vi "FormCalibra5.vi"() -> ()   [LabVIEW 2014]
uses:
  testMachine.ctl
  mainMachine.ctl
  <vilib>/Analysis/baseanly.llb/Mean (DBL).vi
  <vilib>/express/express shared/transition.llb/Dynamic To Waveform Array.vi
  <vilib>/express/express signal manip/GetorSetDDTAttributes/Set DDT Attributes/SetT0.vi
  <vilib>/express/express shared/transition.llb/Waveform Array To Dynamic.vi
  <vilib>/express/express signal manip/GetorSetDDTAttributes/Set DDT Attributes/Set DDT Properties.xnode
  <vilib>/Analysis/NI_AALBase.lvlib
  <resource>/objmgr/daqmx.rc
panel:
  out "deviceName":tag
  out "editTotalWaitLimit":u8
  out "editCountWaitLimit":u8
  out "ledWaitState":bool caption="Wait State"
  out "sliderWaitUpperTime":u8(slide) max=50 scale=0.0..50.0
  out "slideWaitLowerTime":u8(slide) max=30 scale=0.0..30.0
  out "slideWaitTime":u8(slide) scale=0.0..150.0
  out "labelTestTime":string caption="Tempo total de ensaio"
  in  "buttonAcquisition":bool
  in  "editSetWaitTime":u8 caption="Tempo entre ciclos (s)" step=1 format="%0d"
  in  "stop":bool
  out "error out":errorcluster
  out "ledAcquireState":bool caption="Acquire State"
  out "editTotalLowerLimit":u8
  out "editCountLowerLimit":u8
  out "editTotalUpperLimit":u8
  out "editCountUpperLimit":u8
  out "ledEnsaio 3":bool
  out "ledBrakeState":bool caption="Brake State"
  out "ledExitState":bool caption="Exit State"
  out "ledMotorState":bool caption="Motor State"
  out "ledInit2State":bool caption="Init State"
  out "ledBlockState":bool caption="Block State"
  out "ledRunningState":bool caption="Running State"
  out "ledReadyState":bool caption="Ready State"
  out "ledInitState":bool caption="Init State"
  out "mainMachine":T1
  out "testMachine":T2=enum."finish"
  in  "editSetPathToFile":path
  in  "buttonStop":bool
  in  "buttonStart":bool
  out "graphForce":dynamicdata(graph)
  in  "editOffsetForce":dbl caption="Tara" min=0.0 max=100.0 step=0.1
  in  "editSetForce":dbl caption="Fator de conversão"
  out "editForce":dbl caption="Força (Kgf)" format="%#_4f"
  out "graphSpeed":dynamicdata(graph)
  in  "editSetSpeed":dbl caption="Fator de conversão"
  out "editSpeed":dbl caption="Velocidade (km/h)" format="%#_4f"
  out "editEngineSpeed":dbl caption="Rotação (RPM)" format="%#_4f"
  in  "buttonMotor":bool
  in  "buttonBrake":bool
  in  "editSetWaitLowerTime":u8 caption="Tempo de espera (s)"
  in  "editSetWaitUpperTime":u8=3 caption="Tempo de espera (s)"
  in  "editSetNumberOfCycles":u16 caption="Número de ciclos" max=999 step=1 format="%0d"
  in  "editSetLowerLimit":u32 caption="Limite inferior (km/h)"
  in  "editSetUpperLimit":u32 caption="Limite superior (km/h)"
  out "editTempB":dbl caption="Temperatura B (ºC)"
  out "editTempA":dbl caption="Temperatura A (ºC)"
  in  "editSetTempRef":dbl caption="Offset referência" step=0.01 format="%#_2f"
  out "editTempRef":dbl caption="Referência (ºC)"
  out "ledMotor":bool
  out "ledBrake":bool
  out "ledEnsaio":bool
  out "labelTotalCycle":string
  out "labelCurrentCycle":string
  out "labelSystemTitle":string
  in  "editCurrCycleCtr":u32
  in  "velocidade 2":u32
  out "velocidade":u32
  # "Bancada de Frenagem - Ensaio"
  # "Ensaio"
  # "Temperatura"
  # "Rotação"
  # "Célula de Carga"
  # "Configurações do ensaio"
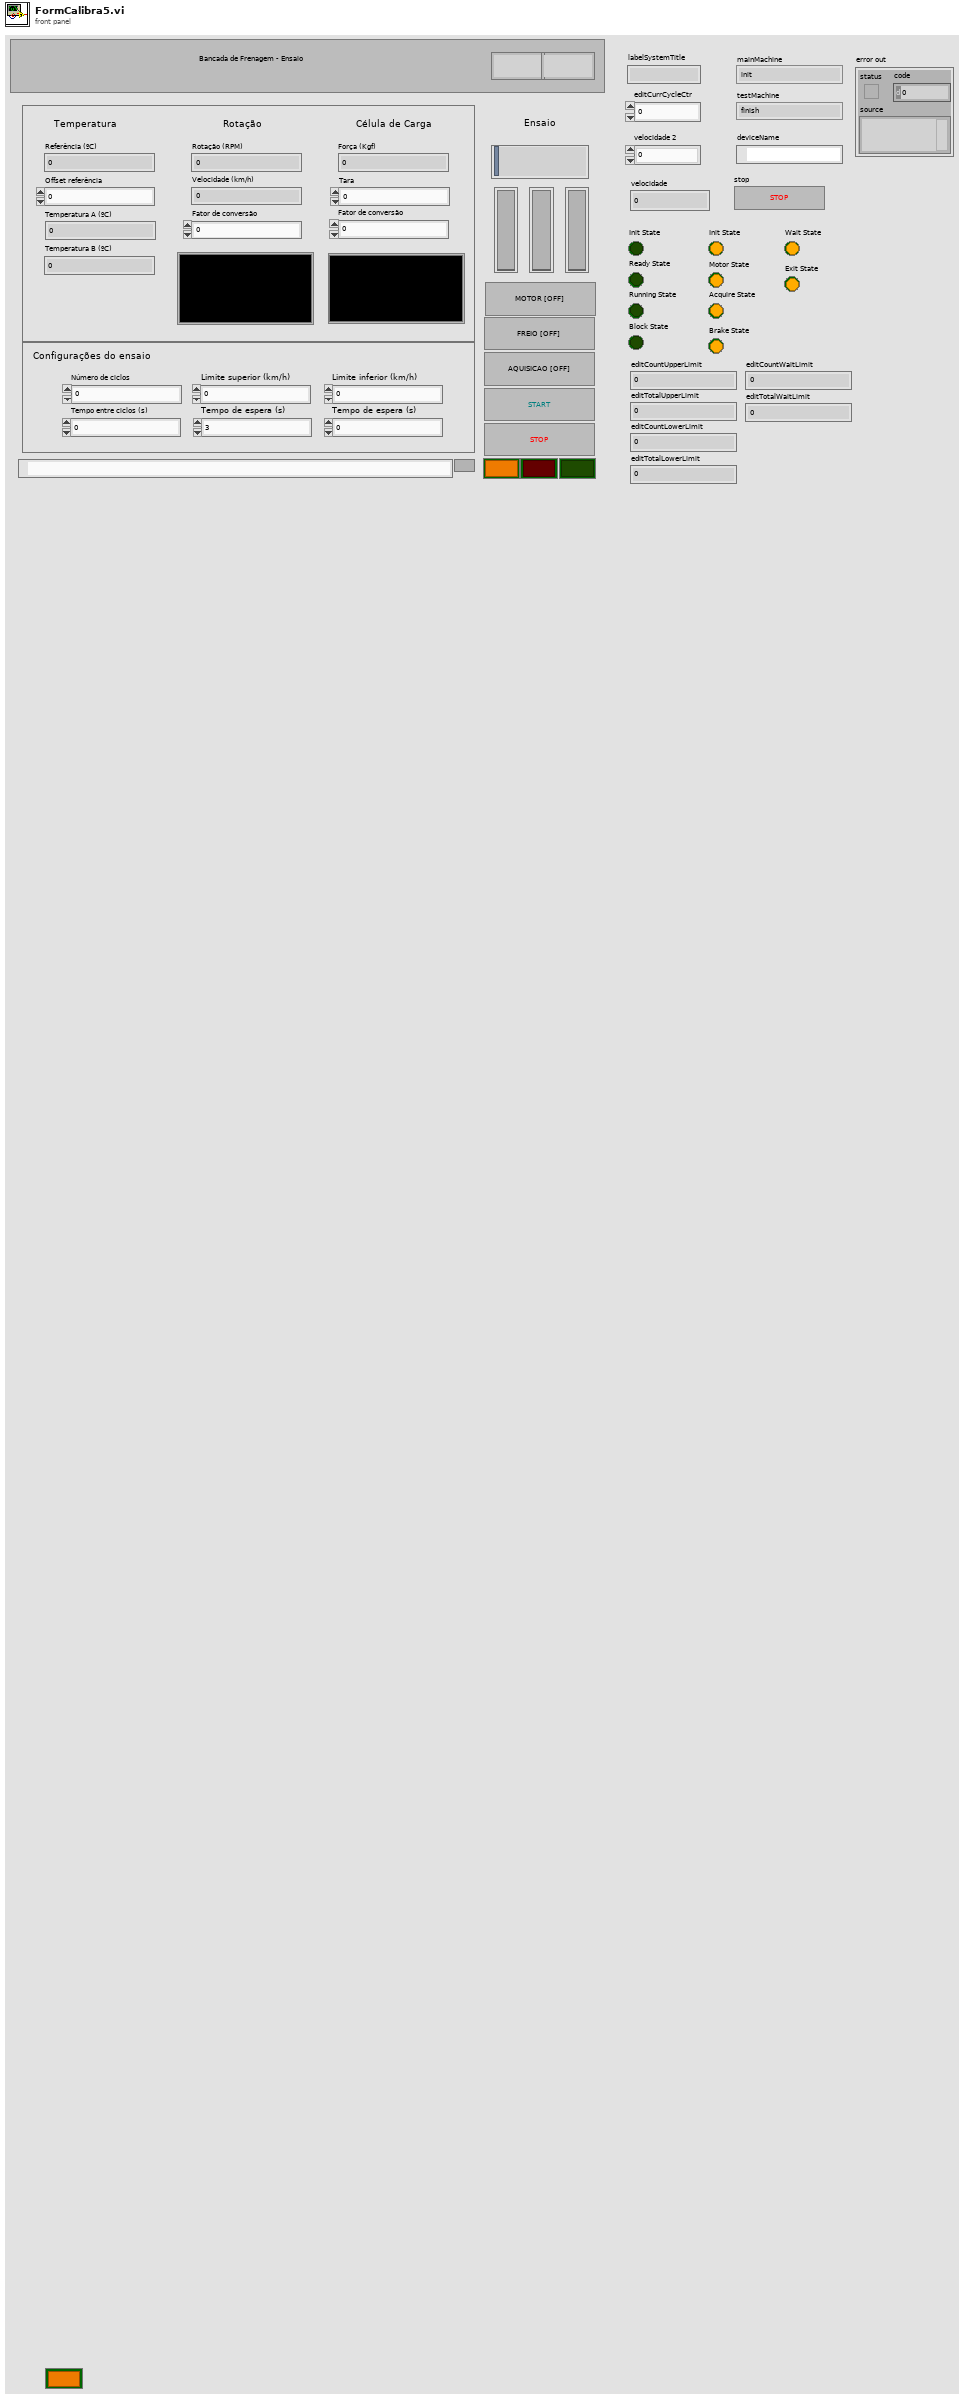
[diagram p1: front panel]
types:
  T1 = typedef "mainMachine.ctl" = enum16{"init", "ready", "running", "blocked", "finish"}
  T2 = typedef "testMachine.ctl" = enum16{"init", "motor", "motor acquire", "brake", "brake acquire", "wait ", "finish", "exit"}
  T3 = enum8{"Enabled", "Disabled", "Disabled and Grayed Out"}
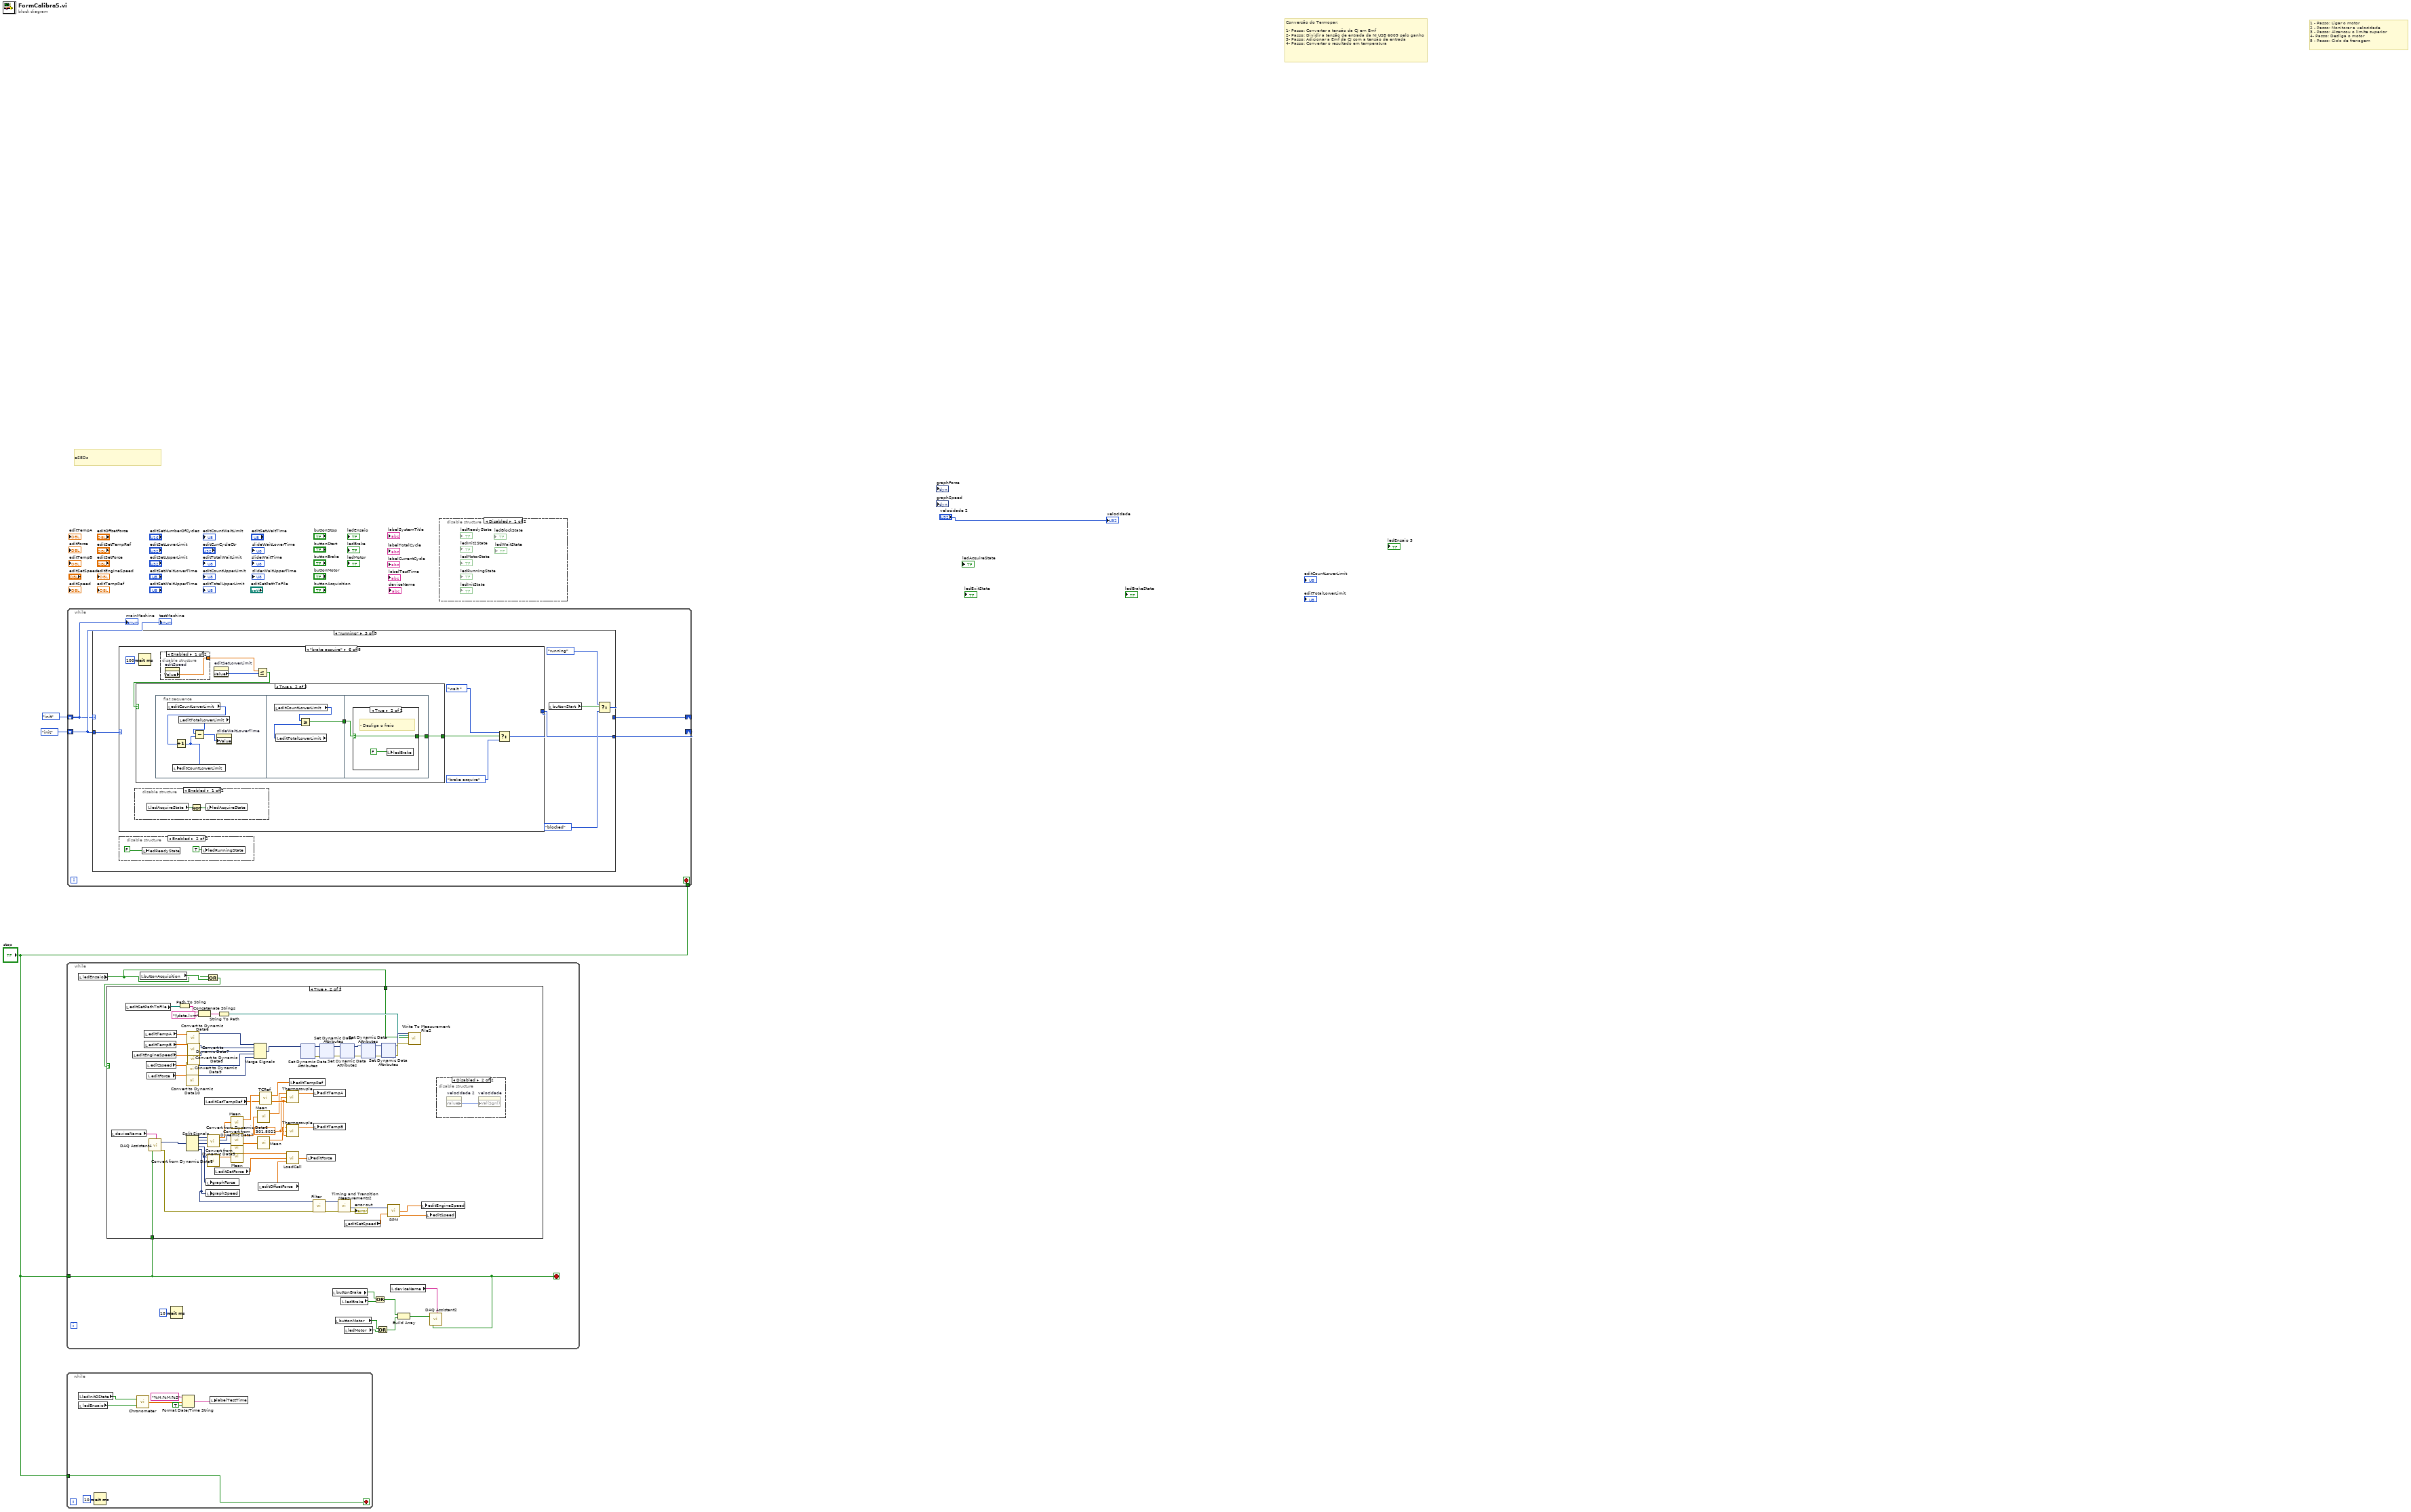
[diagram p0: block diagram]
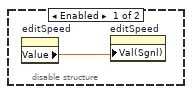
[diagram p4: hidden frame]
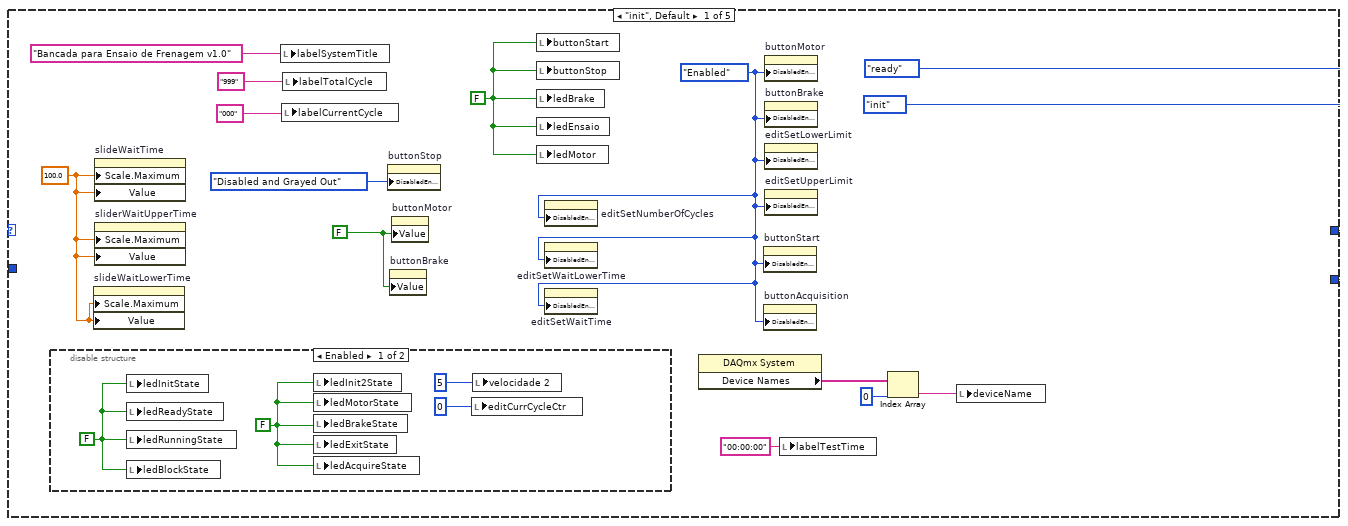
[diagram p5: hidden frame]
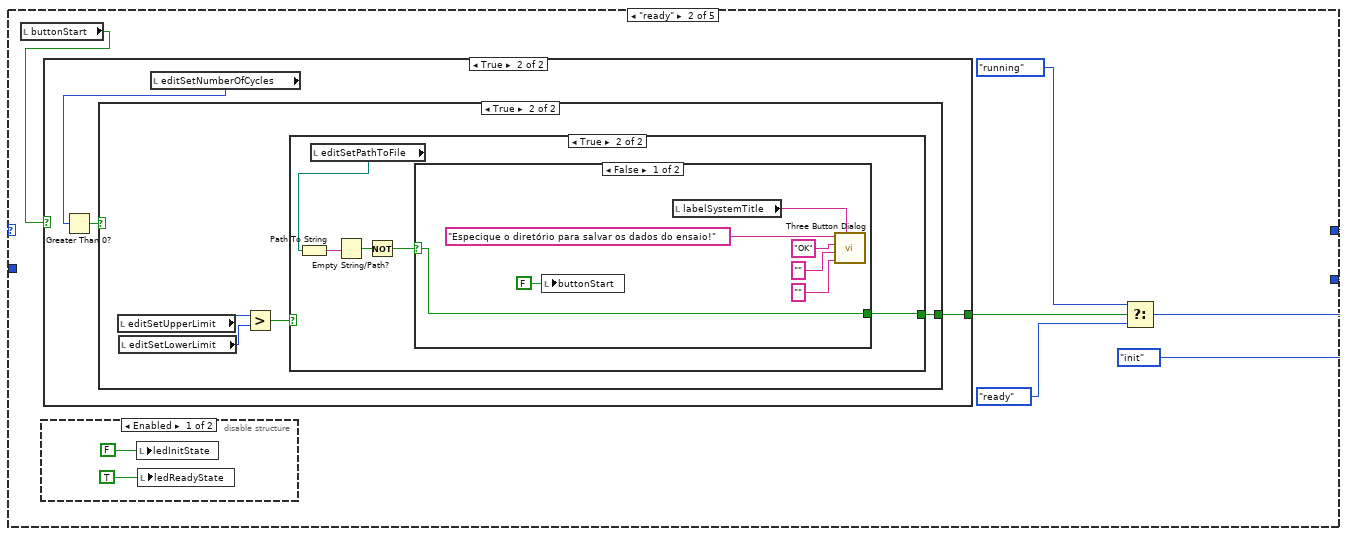
[diagram p7: hidden frame]
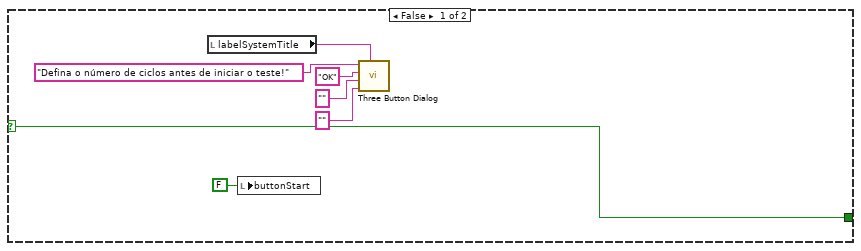
[diagram p10: hidden frame]
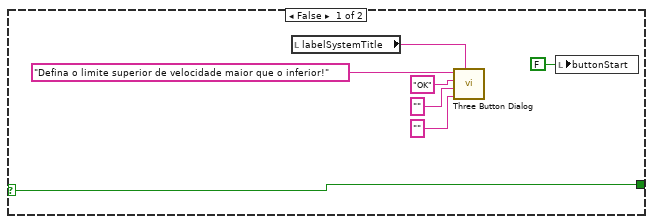
[diagram p11: hidden frame]
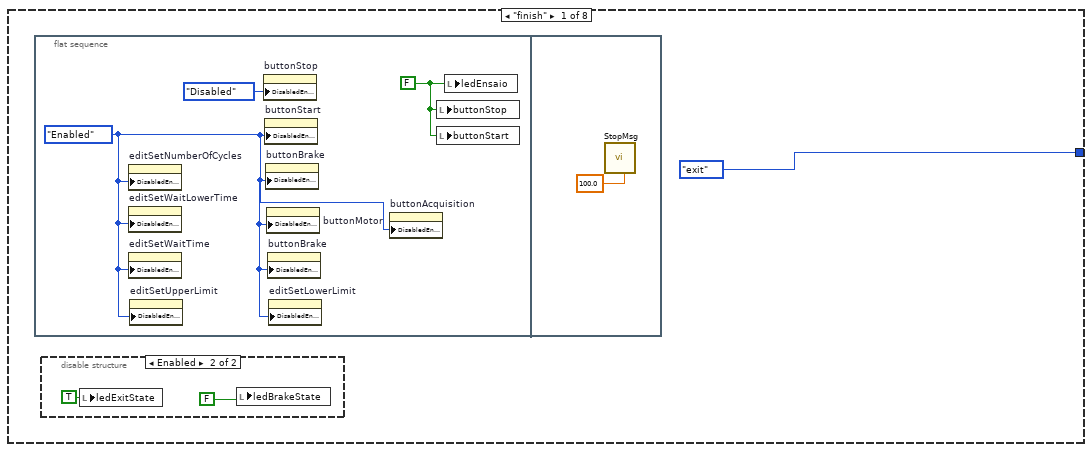
[diagram p14: hidden frame]
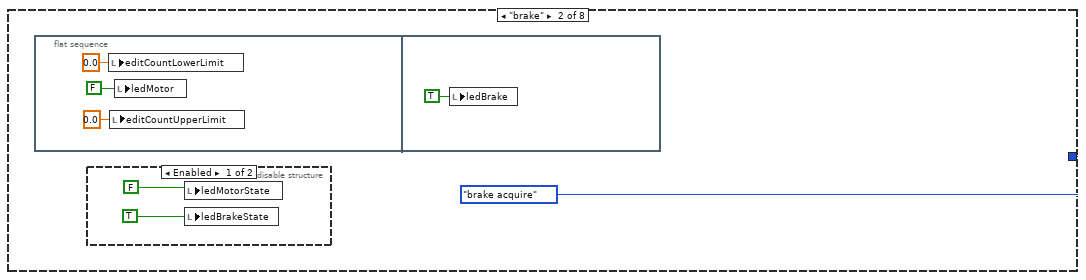
[diagram p16: hidden frame]
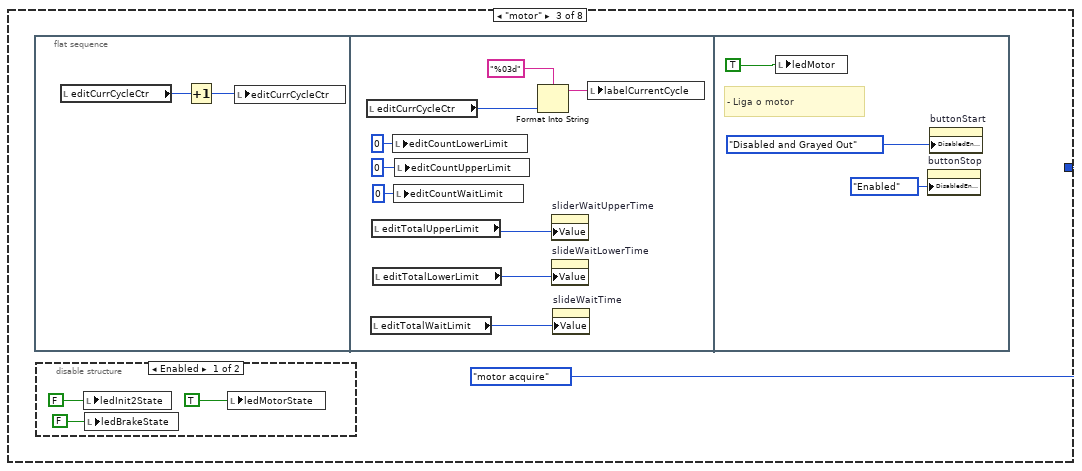
[diagram p18: hidden frame]
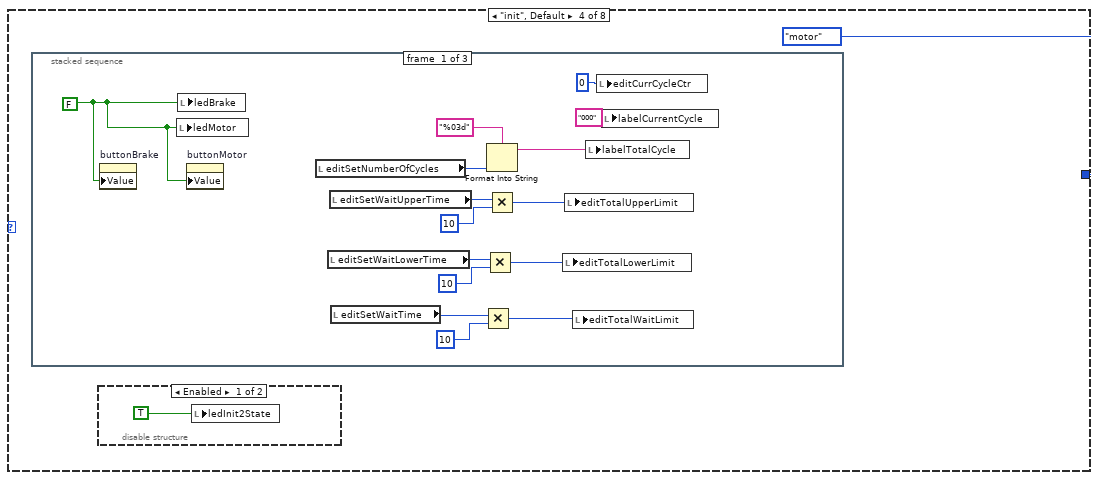
[diagram p20: hidden frame]
diagram:
  # "eSEDs"
  # "1 - Passo: Ligar o motor\n2 - Passo: Monitorar a velocidade\n3 - Passo: Alcancou o limite superior\n4- Passo: Desliga o motor\n5 - Passo: Ciclo de frenagem"
  # "Conversão do Termopar:\n\n1- Passo: Converter a tensão da CJ em Emf\n2- Passo: Dividir a tensão de entrada da NI USB 6009 pelo ganho\n3- Passo: Adicionar a Emf da CJ com a tensão de entrada\n4- Passo: Converter o resultado em temperatura"
  n1 = while {
    tunnel: "stop" -> [w12]
    stop <- w12 stop-if-true
    n2 = local read "ledInit2State"() -> (w6:bool)
    n3 = local read "ledEnsaio"() -> (w5:bool)
    n4 = Wait (ms)(milliseconds to wait=u32 10) -> ()  [unwired: 1 out]
    n5 = call "Chronometer.vi"("start"=w5, "reset"=w6) -> ("Time"=w10:dbl)
    n6 = Format Date/Time String(time format string (%c)="%H:%M:%S", seconds (now)=w10, UTC format=TRUE) -> (date/time string=w7:string)
    n7 = local write "labelTestTime"(w7) -> ()
  }
  n8 = while {
    tunnel: "stop" -> [w18]
    stop <- w18 stop-if-true
    n9 = local read "ledEnsaio"() -> (w15:bool)
    n10 = local read "buttonAcquisition"() -> (w17:bool)
    n11 = Wait (ms)(milliseconds to wait=u32 10) -> ()  [unwired: 1 out]
    n12 = Or(x=w15, y=w17) -> (x .or. y?=w16:bool)
    n13 = case shown="True" w16 {
      tunnel: w18 -> [_ w32]
      tunnel: w15 -> [_ w27]
      frame False {
      }
      frame True {
        w45 = 301.8021 ("factor")
        n14 = local read "deviceName"() -> (w26:tag)
        n15 = local read "editSetPathToFile"() -> (w61:path)
        n16 = local read "editEngineSpeed"() -> (w76:dbl)
        n17 = local read "editTempA"() -> (w73:dbl)
        n18 = local read "editTempB"() -> (w75:dbl)
        n19 = local read "editSpeed"() -> (w77:dbl)
        n20 = local read "editForce"() -> (w78:dbl)
        n21 = call "DAQ Assistant4"("stop (F)"=w32, "device name"=w26) -> ("data"=w34:dynamicdata, "error out"=w30:errorcluster)  [unwired: 14 in, 2 out]
        n22 = Path To String(path=w61) -> (string=w60:string)
        n23 = call "Convert to Dynamic Data9"("Double"=w77) -> ("Dynamic Data Type"=w81:dynamicdata)  [unwired: 3 in]
        n24 = call "Convert to Dynamic Data10"("Double"=w78) -> ("Dynamic Data Type"=w82:dynamicdata)  [unwired: 3 in]
        n25 = Split Signals(w34) -> (w37:dynamicdata, w41:dynamicdata, w39:dynamicdata, w50:dynamicdata, w29:dynamicdata)  [unwired: 5 in]
        n26 = call "Convert to Dynamic Data6"("Double"=w73) -> ("Dynamic Data Type"=w74:dynamicdata)  [unwired: 3 in]
        n27 = call "Convert to Dynamic Data7"("Double"=w75) -> ("Dynamic Data Type"=w79:dynamicdata)  [unwired: 3 in]
        n28 = call "Convert to Dynamic Data8"("Double"=w76) -> ("Dynamic Data Type"=w80:dynamicdata)  [unwired: 3 in]
        n29 = Concatenate Strings(w60, "\\data.lvm" ("string")) -> (w63:string)
        n30 = local read "editSetTempRef"() -> (w36:dbl)
        n31 = local write "graphForce"(w50) -> ()
        n32 = local write "graphSpeed"(w29) -> ()
        n33 = call "Convert from Dynamic Data5"("Dynamic Data Type"=w37) -> ("Array"=w58:dbl[])  [unwired: 3 in]
        n34 = call "Convert from Dynamic Data8"("Dynamic Data Type"=w50) -> ("Array"=w42:dbl[])  [unwired: 3 in]
        n35 = local read "editSetForce"() -> (w56:dbl)
        n36 = String To Path(string=w63) -> (path=w64:path)
        n37 = call-poly <vilib>:"Mean.vi"("X"=w58) -> ("mean"=w59:dbl)  [unwired: 1 out]
        n38 = call "Convert from Dynamic Data6"("Dynamic Data Type"=w41) -> ("Array"=w38:dbl[])  [unwired: 3 in]
        n39 = call "Convert from Dynamic Data7"("Dynamic Data Type"=w39) -> ("Array"=w40:dbl[])  [unwired: 3 in]
        n40 = call-poly <vilib>:"Mean.vi"("X"=w42) -> ("mean"=w49:dbl)  [unwired: 1 out]
        n41 = Merge Signals(w74, w79, w80, w81, w82) -> (w83:dynamicdata)
        n42 = call-poly <vilib>:"Mean.vi"("X"=w38) -> ("mean"=w43:dbl)  [unwired: 1 out]
        n43 = call-poly <vilib>:"Mean.vi"("X"=w40) -> ("mean"=w44:dbl)  [unwired: 1 out]
        n44 = local read "editOffsetForce"() -> (w57:dbl)
        n45 = call "TCRef.vi"("offset"=w36, "data"=w59) -> ("emf(mV)"=w46:dbl, "temp (degC)"=w35:dbl)
        n46 = call "Thermocouple.vi"("cj(mV)"=w46, "factor"=w45, "data"=w43) -> ("temp(degC)"=w47:dbl)  [unwired: 2 out]
        n47 = call "Thermocouple.vi"("cj(mV)"=w46, "factor"=w45, "data"=w44) -> ("temp(degC)"=w48:dbl)  [unwired: 2 out]
        n48 = call "LoadCell.vi"("tara"=w57, "factor"=w56, "data"=w49) -> ("force (Kgf)"=w53:dbl)
        n49 = local write "editTempRef"(w35) -> ()
        n50 = xnode ("Set Dynamic Data Attributes")("Signals In"=w83) -> ("Signals Out"=w65:dynamicdata, "error out"=w67:errorcluster)  [unwired: 4 in]
        n51 = local write "editForce"(w53) -> ()
        n52 = call "Filter"("error in (no error)"=w30, "Signal"=w29) -> ("error out"=w31:errorcluster, "Filtered Signal"=w28:dynamicdata)  [unwired: 8 in]
        n53 = local write "editTempA"(w47) -> ()
        n54 = local write "editTempB"(w48) -> ()
        n55 = xnode ("Set Dynamic Data Attributes")("Signals In"=w65, "error in"=w67) -> ("Signals Out"=w66:dynamicdata, "error out"=w68:errorcluster)  [unwired: 3 in]
        n56 = call "Timing and Transition Measurements2"("error in (no error)"=w31, "Signals"=w28) -> ("error out"=→"error out":errorcluster, "Frequency"=w51:dynamicdata)  [unwired: 8 in]
        n57 = xnode ("Set Dynamic Data Attributes")("Signals In"=w66, "error in"=w68) -> ("Signals Out"=w84:dynamicdata, "error out"=w69:errorcluster)  [unwired: 3 in]
        n58 = local read "editSetSpeed"() -> (w52:dbl)
        n59 = xnode ("Set Dynamic Data Attributes")("Signals In"=w84, "error in"=w69) -> ("Signals Out"=w85:dynamicdata, "error out"=w70:errorcluster)  [unwired: 3 in]
        n60 = xnode ("Set Dynamic Data Attributes")("Signals In"=w85, "error in"=w70) -> ("Signals Out"=w71:dynamicdata, "error out"=w72:errorcluster)  [unwired: 3 in]
        n61 = call "RPM.vi"("data"=w51, "factor"=w52) -> ("RPM"=w54:dbl, "km/h"=w55:dbl)  [unwired: 1 out]
        n62 = call "Write To Measurement File2"("Signals"=w71, "Enable"=w27, "error in (no error)"=w72, "Filename"=w64) -> ()  [unwired: 13 in, 3 out]
        n63 = local write "editEngineSpeed"(w54) -> ()
        n64 = local write "editSpeed"(w55) -> ()
        n65 = disable-structure shown="Disabled" {
          frame Enabled {
            n66 = property on="editSpeed" class="DigNum (strict)"() -> ("Value"=w86:dbl)  [unwired: 2 in, 2 out]
            n67 = property on="editSpeed" class="DigNum (strict)"("Val(Sgnl)"=w86) -> ()  [unwired: 2 in, 2 out]
          }
          frame Disabled {
            n68 = property on="velocidade 2" class="DigNum (strict)"() -> ("Value"=w87:u32)  [unwired: 2 in, 2 out]
            n69 = property on="velocidade" class="DigNum (strict)"("Val(Sgnl)"=w87) -> ()  [unwired: 2 in, 2 out]
          }
        }
      }
    }
    n70 = local read "buttonBrake"() -> (w22:bool)
    n71 = local read "buttonMotor"() -> (w20:bool)
    n72 = local read "ledBrake"() -> (w24:bool)
    n73 = local read "ledMotor"() -> (w21:bool)
    n74 = Or(x=w22, y=w24) -> (x .or. y?=w23:bool)
    n75 = Or(x=w20, y=w21) -> (x .or. y?=w19:bool)
    n76 = local read "deviceName"() -> (w13:tag)
    n77 = Build Array(w23, w19) -> (w25:bool[])
    n78 = call "DAQ Assistant2"("data"=w25, "stop (T)"=w18, "device name"=w13) -> ()  [unwired: 15 in, 2 out]
  }
  n79 = while {
    shift-right: [w182] -> _
    shift-left: mainMachine."init" ("mainMachine") -> [w179]
    shift-right: [w181] -> _
    shift-left: testMachine."init" ("testMachine") -> [w180]
    tunnel: "stop" -> [w178]
    stop <- w178 stop-if-true
    n80 = case shown="\"running\"" w179 {
      tunnel: [mainMachine."ready" ("mainMachine") w201 w246 w386 mainMachine."finish" ("mainMachine")] -> w182
      tunnel: [testMachine."init" ("testMachine") testMachine."init" ("testMachine") w245 testMachine."init" ("testMachine") testMachine."init" ("testMachine")] -> w181
      tunnel: w180 -> [_ _ w244 _ _]
      frame "init", Default {
        w187 = 100.0 ("Scale.Range:Maximum")
        w188 = T3."Enabled" ("Disabled")
        w189 = FALSE ("buttonMotor")
        w195 = FALSE ("motor")
        n81 = disable-structure shown="Enabled" {
          frame Enabled {
            w197 = FALSE
            w198 = FALSE
            n82 = local write "ledInitState"(w198) -> ()
            n83 = local write "ledReadyState"(w198) -> ()
            n84 = local write "ledRunningState"(w198) -> ()
            n85 = local write "ledBlockState"(w198) -> ()
            n86 = local write "ledInit2State"(w197) -> ()
            n87 = local write "ledMotorState"(w197) -> ()
            n88 = local write "ledBrakeState"(w197) -> ()
            n89 = local write "ledExitState"(w197) -> ()
            n90 = local write "ledAcquireState"(w197) -> ()
            n91 = local write "editCurrCycleCtr"(u32 0 ("currentCycleCtr")) -> ()
            n92 = local write "velocidade 2"(u32 5 ("velocidade 2")) -> ()
          }
          frame Disabled {
          }
        }
        n93 = property on="slideWaitLowerTime" class="Slide (strict)"("Scale.Maximum"=w187, "Value"=w187) -> ()  [unwired: 2 in, 2 out]
        n94 = property on="slideWaitTime" class="Slide (strict)"("Scale.Maximum"=w187, "Value"=w187) -> ()  [unwired: 2 in, 2 out]
        n95 = property on="sliderWaitUpperTime" class="Slide (strict)"("Scale.Maximum"=w187, "Value"=w187) -> ()  [unwired: 2 in, 2 out]
        n96 = local write "labelSystemTitle"("Bancada para Ensaio de Frenagem v1.0" ("systemTitle")) -> ()
        n97 = local write "labelCurrentCycle"("000" ("currentCycle")) -> ()
        n98 = local write "labelTotalCycle"("999" ("totalCycle")) -> ()
        n99 = property on="buttonStop" class="Bool (strict)"("DisabledEnum"=T3."Disabled and Grayed Out" ("Disabled")) -> ()  [unwired: 2 in, 2 out]
        n100 = property on="buttonBrake" class="Bool (strict)"("Value"=w189) -> ()  [unwired: 2 in, 2 out]
        n101 = property on="buttonMotor" class="Bool (strict)"("Value"=w189) -> ()  [unwired: 2 in, 2 out]
        n102 = local write "buttonStart"(w195) -> ()
        n103 = local write "buttonStop"(w195) -> ()
        n104 = local write "ledBrake"(w195) -> ()
        n105 = local write "ledEnsaio"(w195) -> ()
        n106 = local write "ledMotor"(w195) -> ()
        n107 = property on="editSetNumberOfCycles" class="DigNum (strict)"("DisabledEnum"=w188) -> ()  [unwired: 2 in, 2 out]
        n108 = property on="editSetWaitLowerTime" class="DigNum (strict)"("DisabledEnum"=w188) -> ()  [unwired: 2 in, 2 out]
        n109 = property on="editSetWaitTime" class="DigNum (strict)"("DisabledEnum"=w188) -> ()  [unwired: 2 in, 2 out]
        n110 = property class="DAQmx System"() -> ("Device Names"=w186:tag[])  [unwired: 2 in, 2 out]
        n111 = property on="buttonStart" class="Bool (strict)"("DisabledEnum"=w188) -> ()  [unwired: 2 in, 2 out]
        n112 = property on="buttonAcquisition" class="Bool (strict)"("DisabledEnum"=w188) -> ()  [unwired: 2 in, 2 out]
        n113 = property on="buttonMotor" class="Bool (strict)"("DisabledEnum"=w188) -> ()  [unwired: 2 in, 2 out]
        n114 = property on="buttonBrake" class="Bool (strict)"("DisabledEnum"=w188) -> ()  [unwired: 2 in, 2 out]
        n115 = property on="editSetLowerLimit" class="DigNum (strict)"("DisabledEnum"=w188) -> ()  [unwired: 2 in, 2 out]
        n116 = property on="editSetUpperLimit" class="DigNum (strict)"("DisabledEnum"=w188) -> ()  [unwired: 2 in, 2 out]
        n117 = local write "labelTestTime"("00:00:00" ("labelTestTime")) -> ()
        n118 = Index Array(array=w186, index=0) -> (element=w184:tag)
        n119 = local write "deviceName"(w184) -> ()
      }
      frame "ready" {
        n120 = local read "buttonStart"() -> (w204:bool)
        n121 = disable-structure shown="Enabled" {
          frame Enabled {
            n122 = local write "ledInitState"(FALSE ("ledReady")) -> ()
            n123 = local write "ledReadyState"(TRUE ("ledReady")) -> ()
          }
          frame Disabled {
          }
        }
        n124 = case shown="True" w204 {
          selector: w204 -> [w209 _]
          tunnel: [w209 w210] -> w203
          frame False {
          }
          frame True {
            n125 = local read "editSetNumberOfCycles"() -> (w211:u16)
            n126 = Greater Than 0?(x=w211) -> (x > 0?=w212:bool)
            n127 = case shown="True" w212 {
              selector: w212 -> [w219 _]
              tunnel: [w219 w220] -> w210
              frame False {
                n128 = local read "labelSystemTitle"() -> (w214:string)
                n129 = local write "buttonStart"(FALSE ("startButton")) -> ()
                n130 = call <vilib>:"Three Button Dialog.vi"("Window Title (\"\")"=w214, "Right Button Text (\"Cancel\")"="" ("Right Button Text (\"Cancel\")"), "Center Button Text (\"No\")"="" ("Center Button Text (\"No\")"), "Left Button Text (\"Yes\")"="OK" ("Left Button Text (\"Yes\")"), "message"="Defina o número de ciclos antes de iniciar o teste!") -> ()  [unwired: 6 in, 1 out]
              }
              frame True {
                n131 = local read "editSetUpperLimit"() -> (w222:u32)
                n132 = local read "editSetLowerLimit"() -> (w221:u32)
                n133 = Greater?(x=w222, y=w221) -> (0:w223:bool)
                n134 = case shown="True" w223 {
                  selector: w223 -> [w230 _]
                  tunnel: [w230 w233] -> w220
                  frame False {
                    n135 = local read "labelSystemTitle"() -> (w225:string)
                    n136 = call <vilib>:"Three Button Dialog.vi"("Window Title (\"\")"=w225, "Right Button Text (\"Cancel\")"="" ("Right Button Text (\"Cancel\")"), "Center Button Text (\"No\")"="" ("Center Button Text (\"No\")"), "Left Button Text (\"Yes\")"="OK" ("Left Button Text (\"Yes\")"), "message"="Defina o limite superior de velocidade maior que o inferior!") -> ()  [unwired: 6 in, 1 out]
                    n137 = local write "buttonStart"(FALSE ("startButton")) -> ()
                  }
                  frame True {
                    n138 = local read "editSetPathToFile"() -> (w235:path)
                    n139 = Path To String(path=w235) -> (string=w234:string)
                    n140 = Empty String/Path?(string/path=w234) -> (empty?=w232:bool)
                    n141 = Not(x=w232) -> (.not. x?=w231:bool)
                    n142 = case shown="False" w231 {
                      selector: w231 -> [w242 w243]
                      tunnel: [w242 w243] -> w233
                      frame False {
                        n143 = local write "buttonStart"(FALSE ("startButton")) -> ()
                        n144 = local read "labelSystemTitle"() -> (w237:string)
                        n145 = call <vilib>:"Three Button Dialog.vi"("Window Title (\"\")"=w237, "Right Button Text (\"Cancel\")"="" ("Right Button Text (\"Cancel\")"), "Center Button Text (\"No\")"="" ("Center Button Text (\"No\")"), "Left Button Text (\"Yes\")"="OK" ("Left Button Text (\"Yes\")"), "message"="Especique o diretório para salvar os dados do ensaio!") -> ()  [unwired: 6 in, 1 out]
                      }
                      frame True {
                      }
                    }
                  }
                }
              }
            }
          }
        }
        n146 = Select(t=mainMachine."running" ("mainMachine"), s=w203, f=mainMachine."ready" ("mainMachine")) -> (s? t:f=w201:T1)
      }
      frame "running" {
        n147 = case shown="\"brake acquire\"" w244 {
          tunnel: [testMachine."exit" ("testMachine") testMachine."brake acquire" ("testMachine") testMachine."motor acquire" ("testMachine") testMachine."motor" ("testMachine") w316 w336 testMachine."exit" ("testMachine") w369] -> w245
          frame "finish" {
            n148 = flat-sequence {
              frame #0 {
                w256 = FALSE ("ledReady")
                w255 = T3."Enabled" ("Disabled")
                n149 = property on="editSetNumberOfCycles" class="DigNum (strict)"("DisabledEnum"=w255) -> ()  [unwired: 2 in, 2 out]
                n150 = property on="editSetWaitLowerTime" class="DigNum (strict)"("DisabledEnum"=w255) -> ()  [unwired: 2 in, 2 out]
                n151 = property on="editSetWaitTime" class="DigNum (strict)"("DisabledEnum"=w255) -> ()  [unwired: 2 in, 2 out]
                n152 = property on="editSetUpperLimit" class="DigNum (strict)"("DisabledEnum"=w255) -> ()  [unwired: 2 in, 2 out]
                n153 = property on="buttonStop" class="Bool (strict)"("DisabledEnum"=T3."Disabled" ("Disabled")) -> ()  [unwired: 2 in, 2 out]
                n154 = property on="buttonStart" class="Bool (strict)"("DisabledEnum"=w255) -> ()  [unwired: 2 in, 2 out]
                n155 = property on="buttonBrake" class="Bool (strict)"("DisabledEnum"=w255) -> ()  [unwired: 2 in, 2 out]
                n156 = property on="buttonMotor" class="Bool (strict)"("DisabledEnum"=w255) -> ()  [unwired: 2 in, 2 out]
                n157 = property on="buttonBrake" class="Bool (strict)"("DisabledEnum"=w255) -> ()  [unwired: 2 in, 2 out]
                n158 = property on="editSetLowerLimit" class="DigNum (strict)"("DisabledEnum"=w255) -> ()  [unwired: 2 in, 2 out]
                n159 = property on="buttonAcquisition" class="Bool (strict)"("DisabledEnum"=w255) -> ()  [unwired: 2 in, 2 out]
                n160 = local write "buttonStop"(w256) -> ()
                n161 = local write "buttonStart"(w256) -> ()
                n162 = local write "ledEnsaio"(w256) -> ()
              }
              frame #1 {
                n163 = call "StopMsg.vi"("Max Value (100)"=100.0) -> ()  [unwired: 8 in, 2 out]
              }
            }
            n164 = disable-structure shown="Enabled" {
              frame Disabled {
              }
              frame Enabled {
                n165 = local write "ledExitState"(TRUE ("ledReady")) -> ()
                n166 = local write "ledBrakeState"(FALSE ("ledReady")) -> ()
              }
            }
          }
          frame "brake" {
            n167 = flat-sequence {
              frame #0 {
                n168 = local write "editCountLowerLimit"(0.0 ("editCountUpperLimit")) -> ()
                n169 = local write "editCountUpperLimit"(0.0 ("editCountUpperLimit")) -> ()
                n170 = local write "ledMotor"(FALSE ("motor")) -> ()
              }
              frame #1 {
                n171 = local write "ledBrake"(TRUE ("freio")) -> ()
              }
            }
            n172 = disable-structure shown="Enabled" {
              frame Enabled {
                n173 = local write "ledMotorState"(FALSE ("ledReady")) -> ()
                n174 = local write "ledBrakeState"(TRUE ("ledReady")) -> ()
              }
              frame Disabled {
              }
            }
          }
          frame "motor" {
            n175 = flat-sequence {
              frame #0 {
                n176 = local read "editCurrCycleCtr"() -> (w271:u32)
                n177 = Increment(x=w271) -> (x+1=w270:u32)
                n178 = local write "editCurrCycleCtr"(w270) -> ()
              }
              frame #1 {
                n179 = local read "editCurrCycleCtr"() -> (w278:u32)
                n180 = local read "editTotalWaitLimit"() -> (w272:u8)
                n181 = local read "editTotalUpperLimit"() -> (w274:u8)
                n182 = local read "editTotalLowerLimit"() -> (w273:u8)
                n183 = local write "editCountLowerLimit"(u8 0 ("editCountLowerLimit")) -> ()
                n184 = local write "editCountWaitLimit"(u8 0 ("editCountWaitLimit")) -> ()
                n185 = local write "editCountUpperLimit"(u8 0 ("editCountUpperLimit")) -> ()
                n186 = Format Into String(format string="%03d", w278) -> (resulting string=w279:string)  [unwired: 2 in, 1 out]
                n187 = property on="sliderWaitUpperTime" class="Slide (strict)"("Value"=w274) -> ()  [unwired: 2 in, 2 out]
                n188 = property on="slideWaitLowerTime" class="Slide (strict)"("Value"=w273) -> ()  [unwired: 2 in, 2 out]
                n189 = property on="slideWaitTime" class="Slide (strict)"("Value"=w272) -> ()  [unwired: 2 in, 2 out]
                n190 = local write "labelCurrentCycle"(w279) -> ()
              }
              frame #2 {
                # "- Liga o motor"
                n191 = local write "ledMotor"(TRUE ("motor")) -> ()
                n192 = property on="buttonStop" class="Bool (strict)"("DisabledEnum"=T3."Enabled" ("Disabled")) -> ()  [unwired: 2 in, 2 out]
                n193 = property on="buttonStart" class="Bool (strict)"("DisabledEnum"=T3."Disabled and Grayed Out" ("Disabled")) -> ()  [unwired: 2 in, 2 out]
              }
            }
            n194 = disable-structure shown="Enabled" {
              frame Enabled {
                n195 = local write "ledInit2State"(FALSE ("ledReady")) -> ()
                n196 = local write "ledBrakeState"(FALSE ("ledReady")) -> ()
                n197 = local write "ledMotorState"(TRUE ("ledReady")) -> ()
              }
              frame Disabled {
              }
            }
          }
          frame "init", Default {
            n198 = stacked-sequence {
              frame #0 {
                w291 = FALSE ("ensaio")
                n199 = property on="buttonBrake" class="Bool (strict)"("Value"=w291) -> ()  [unwired: 2 in, 2 out]
                n200 = local write "ledMotor"(w291) -> ()
                n201 = local write "ledBrake"(w291) -> ()
                n202 = property on="buttonMotor" class="Bool (strict)"("Value"=w291) -> ()  [unwired: 2 in, 2 out]
                n203 = local read "editSetNumberOfCycles"() -> (w298:u16)
                n204 = local read "editSetWaitLowerTime"() -> (w292:u8)
                n205 = local read "editSetWaitUpperTime"() -> (w295:u8)
                n206 = local read "editSetWaitTime"() -> (w286:u8)
                n207 = Multiply(x=w286, y=u32 10) -> (x*y=w287:u32)
                n208 = Multiply(x=w292, y=u32 10) -> (x*y=w290:u32)
                n209 = Format Into String(format string="%03d", w298) -> (resulting string=w299:string)  [unwired: 2 in, 1 out]
                n210 = Multiply(x=w295, y=u32 10) -> (x*y=w289:u32)
                n211 = local write "editTotalLowerLimit"(w290) -> ()
                n212 = local write "editTotalUpperLimit"(w289) -> ()
                n213 = local write "editTotalWaitLimit"(w287) -> ()
                n214 = local write "labelTotalCycle"(w299) -> ()
                n215 = local write "editCurrCycleCtr"(u32 0 ("currentCycleCtr")) -> ()
                n216 = local write "labelCurrentCycle"("000" ("currentCycle")) -> ()
              }
              frame #1 {
                w307 = T3."Disabled" ("Disabled")
                n217 = property on="editSetNumberOfCycles" class="DigNum (strict)"("DisabledEnum"=w307) -> ()  [unwired: 2 in, 2 out]
                n218 = property on="editSetWaitLowerTime" class="DigNum (strict)"("DisabledEnum"=w307) -> ()  [unwired: 2 in, 2 out]
                n219 = property on="editSetWaitTime" class="DigNum (strict)"("DisabledEnum"=w307) -> ()  [unwired: 2 in, 2 out]
                n220 = local read "editTotalUpperLimit"() -> (w310:u8)
                n221 = property on="sliderWaitUpperTime" class="Slide (strict)"("Scale.Maximum"=w310, "Scale.Minimum"=0.0 ("Scale.Range:Minimum"), "Scale.Increment"=1.0 ("Scale.Range:Increment"), "Value"=w310) -> ()  [unwired: 2 in, 2 out]
                n222 = property on="buttonAcquisition" class="Bool (strict)"("DisabledEnum"=w307) -> ()  [unwired: 2 in, 2 out]
                n223 = local read "editTotalLowerLimit"() -> (w304:u8)
                n224 = property on="slideWaitLowerTime" class="Slide (strict)"("Scale.Maximum"=w304, "Scale.Minimum"=0.0 ("Scale.Range:Minimum"), "Scale.Increment"=1.0 ("Scale.Range:Increment"), "Value"=w304) -> ()  [unwired: 2 in, 2 out]
                n225 = local read "editTotalWaitLimit"() -> (w301:u8)
                n226 = property on="slideWaitTime" class="Slide (strict)"("Scale.Maximum"=w301, "Scale.Minimum"=0.0 ("Scale.Range:Minimum"), "Scale.Increment"=1.0 ("Scale.Range:Increment"), "Value"=w301) -> ()  [unwired: 2 in, 2 out]
                n227 = call "StarMsg.vi"("Show"=TRUE, "Max Value (100)"=100.0) -> ()  [unwired: 7 in, 2 out]
                n228 = property on="buttonMotor" class="Bool (strict)"("DisabledEnum"=w307) -> ()  [unwired: 2 in, 2 out]
                n229 = property on="buttonBrake" class="Bool (strict)"("DisabledEnum"=w307) -> ()  [unwired: 2 in, 2 out]
                n230 = property on="editSetLowerLimit" class="DigNum (strict)"("DisabledEnum"=w307) -> ()  [unwired: 2 in, 2 out]
                n231 = property on="editSetUpperLimit" class="DigNum (strict)"("DisabledEnum"=w307) -> ()  [unwired: 2 in, 2 out]
              }
              frame #2 {
                n232 = local write "ledEnsaio"(TRUE ("ensaio")) -> ()
              }
            }
            n233 = disable-structure shown="Enabled" {
              frame Enabled {
                n234 = local write "ledInit2State"(TRUE ("ledReady")) -> ()
              }
              frame Disabled {
              }
            }
          }
          frame "motor acquire" {
            n235 = disable-structure shown="Enabled" {
              frame Enabled {
                n236 = local read "ledAcquireState"() -> (w325:bool)
                n237 = Not(x=w325) -> (.not. x?=w324:bool)
                n238 = local write "ledAcquireState"(w324) -> ()
              }
              frame Disabled {
              }
            }
            n239 = Wait (ms)(milliseconds to wait=u32 100) -> ()  [unwired: 1 out]
            n240 = disable-structure shown="Enabled" {
              disable-tunnel: [w322 w323] -> w315
              frame Enabled {
                n241 = property on="editSpeed" class="DigNum (strict)"() -> ("Value"=w322:dbl)  [unwired: 2 in, 2 out]
              }
              frame Disabled {
                n242 = property on="velocidade" class="DigNum (strict)"() -> ("Value"=w323:u32)  [unwired: 2 in, 2 out]
              }
            }
            n243 = property on="editSetUpperLimit" class="DigNum (strict)"() -> ("Value"=w314:u32)  [unwired: 2 in, 2 out]
            n244 = Greater Or Equal?(x=w315, y=w314) -> (x >= y?=w320:bool)
            n245 = case shown="True" w320 {
              selector: w320 -> [w326 _]
              tunnel: [w326 w327] -> w319
              frame False {
              }
              frame True {
                n246 = flat-sequence {
                  tunnel: [w332] -> w327
                  frame #0 {
                    n247 = local read "editCountUpperLimit"() -> (w330:u8)
                    n248 = Increment(x=w330) -> (x+1=w328:u8)
                    n249 = local write "editCountUpperLimit"(w328) -> ()
                    n250 = local read "editTotalUpperLimit"() -> (w329:u8)
                    n251 = Subtract(x=w329, y=w328) -> (x-y=w331:u8)
                    n252 = property on="sliderWaitUpperTime" class="Slide (strict)"("Value"=w331) -> ()  [unwired: 2 in, 2 out]
                  }
                  frame #1 {
                    n253 = local read "editCountUpperLimit"() -> (w334:u8)
                    n254 = local read "editTotalUpperLimit"() -> (w333:u8)
                    n255 = Greater Or Equal?(x=w334, y=w333) -> (x >= y?=w332:bool)
                  }
                }
              }
            }
            n256 = Select(t=testMachine."brake" ("testMachine"), s=w319, f=testMachine."motor acquire" ("testMachine")) -> (s? t:f=w316:T2)
          }
          frame "brake acquire" {
            n257 = disable-structure shown="Enabled" {
              frame Enabled {
                n258 = local read "ledAcquireState"() -> (w344:bool)
                n259 = Not(x=w344) -> (.not. x?=w343:bool)
                n260 = local write "ledAcquireState"(w343) -> ()
              }
              frame Disabled {
              }
            }
            n261 = Wait (ms)(milliseconds to wait=u32 100) -> ()  [unwired: 1 out]
            n262 = disable-structure shown="Enabled" {
              disable-tunnel: [w345 w346] -> w335
              frame Enabled {
                n263 = property on="editSpeed" class="DigNum (strict)"() -> ("Value"=w345:dbl)  [unwired: 2 in, 2 out]
              }
              frame Disabled {
                n264 = property on="velocidade" class="DigNum (strict)"() -> ("Value"=w346:u32)  [unwired: 2 in, 2 out]
              }
            }
            n265 = property on="editSetLowerLimit" class="DigNum (strict)"() -> ("Value"=w337:u32)  [unwired: 2 in, 2 out]
            n266 = Less Or Equal?(x=w335, y=w337) -> (x <= y?=w341:bool)
            n267 = case shown="True" w341 {
              selector: w341 -> [w347 _]
              tunnel: [w347 w348] -> w339
              frame False {
              }
              frame True {
                n268 = flat-sequence {
                  tunnel: [w354] -> w349
                  tunnel: w349 -> [w358]
                  tunnel: [w357] -> w348
                  frame #0 {
                    n269 = local read "editCountLowerLimit"() -> (w353:u8)
                    n270 = Increment(x=w353) -> (x+1=w352:u8)
                    n271 = local write "editCountLowerLimit"(w352) -> ()
                    n272 = local read "editTotalLowerLimit"() -> (w351:u8)
                    n273 = Subtract(x=w351, y=w352) -> (x-y=w350:u8)
                    n274 = property on="slideWaitLowerTime" class="Slide (strict)"("Value"=w350) -> ()  [unwired: 2 in, 2 out]
                  }
                  frame #1 {
                    n275 = local read "editCountLowerLimit"() -> (w356:u8)
                    n276 = local read "editTotalLowerLimit"() -> (w355:u8)
                    n277 = Greater Or Equal?(x=w356, y=w355) -> (x >= y?=w354:bool)
                  }
                  frame #2 {
                    n278 = case shown="True" w358 {
                      selector: w358 -> [w359 w360]
                      tunnel: [w359 w360] -> w357
                      frame False {
                      }
                      frame True {
                        # "- Desliga o freio"
                        n279 = local write "ledBrake"(FALSE ("freio")) -> ()
                      }
                    }
                  }
                }
              }
            }
            n280 = Select(t=testMachine."wait " ("testMachine"), s=w339, f=testMachine."brake acquire" ("testMachine")) -> (s? t:f=w336:T2)
          }
          frame "exit" {
          }
          frame "wait " {
            # "- Aguarda 0.5s \n- Atualiza o numero de ciclos"
            n281 = flat-sequence {
              tunnel: [w375] -> w363
              frame #0 {
                n282 = local read "editCountWaitLimit"() -> (w371:u8)
                n283 = Increment(x=w371) -> (x+1=w372:u8)
                n284 = local write "editCountWaitLimit"(w372) -> ()
                n285 = local read "editTotalWaitLimit"() -> (w374:u8)
                n286 = Subtract(x=w374, y=w372) -> (x-y=w373:u8)
                n287 = property on="slideWaitTime" class="Slide (strict)"("Value"=w373) -> ()  [unwired: 2 in, 2 out]
              }
              frame #1 {
                n288 = local read "editCountWaitLimit"() -> (w377:u8)
                n289 = local read "editTotalWaitLimit"() -> (w376:u8)
                n290 = Greater Or Equal?(x=w377, y=w376) -> (x >= y?=w375:bool)
              }
            }
            n291 = disable-structure shown="Enabled" {
              frame Enabled {
                n292 = local read "ledWaitState"() -> (w384:bool)
                n293 = Not(x=w384) -> (.not. x?=w383:bool)
                n294 = local write "ledBrakeState"(FALSE ("ledBrakeState")) -> ()
                n295 = local write "ledWaitState"(w383) -> ()
              }
              frame Disabled {
              }
            }
            n296 = Wait (ms)(milliseconds to wait=u32 100) -> ()  [unwired: 1 out]
            n297 = case shown="True" w363 {
              selector: w363 -> [w378 _]
              tunnel: [w378 w382] -> w364
              frame False {
              }
              frame True {
                n298 = local read "editSetNumberOfCycles"() -> (w380:u16)
                n299 = local read "editCurrCycleCtr"() -> (w379:u32)
                n300 = Greater Or Equal?(x=w379, y=w380) -> (x >= y?=w382:bool)
                n301 = Not(x=w382) -> (.not. x?=w381:bool)
                n302 = local write "ledEnsaio"(w381) -> ()
              }
            }
            n303 = Select(t=testMachine."motor" ("testMachine"), s=w363, f=testMachine."wait " ("testMachine")) -> (s? t:f=w365:T2)
            n304 = Select(t=testMachine."finish" ("testMachine"), s=w364, f=w365) -> (s? t:f=w369:T2)
          }
        }
        n305 = disable-structure shown="Enabled" {
          frame Disabled {
          }
          frame Enabled {
            n306 = local write "ledReadyState"(FALSE ("ledReady")) -> ()
            n307 = local write "ledRunningState"(TRUE ("ledReady")) -> ()
          }
        }
        n308 = local read "buttonStart"() -> (w249:bool)
        n309 = Select(t=mainMachine."running" ("mainMachine"), s=w249, f=mainMachine."blocked" ("mainMachine")) -> (s? t:f=w246:T1)
      }
      frame "blocked" {
        n310 = local read "buttonStart"() -> (w390:bool)
        n311 = Select(t=mainMachine."ready" ("mainMachine"), s=w390, f=mainMachine."blocked" ("mainMachine")) -> (s? t:f=w386:T1)
        n312 = local write "ledRunningState"(FALSE ("ledReady")) -> ()
        n313 = local write "ledBlockState"(TRUE ("ledReady")) -> ()
      }
      frame "finish" {
        n314 = local write "ledBlockState"(FALSE ("ledReady")) -> ()
      }
    }
    "mainMachine" <- w179
    "testMachine" <- w180
  }
  n315 = disable-structure shown="Disabled" {
    frame Disabled {
    }
    frame Enabled {
    }
  }
  "velocidade" <- "velocidade 2"
